vi "Zero Phase Lowpass Filter.vi"   [LabVIEW 2019, in "xy_utilities.lvlib"]
doc: "Apply a Zero Phase Lowpass Filter to <b>XY-Data<b/>'s Y-Array.\n\n<b>cutoff period</b> is equivalent to 1/cutoff frequency and is in the units of the X-Array. The cutoff frequency is restricted between 0 and Fs/4.\n\nWire data to the data input to determine the polymorphic instance to use or manually select the instance."
uses:
  xy_utilities.lvlib
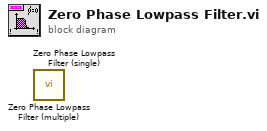
[diagram p0: block diagram]
diagram:
  n1 = call "Zero Phase Lowpass Filter (multiple).vi"() -> ()  [unwired: 10 in, 2 out]
  n2 = call "Zero Phase Lowpass Filter (single).vi"() -> ()  [unwired: 10 in, 2 out]
